vi "Interpret Q Size.vi"(7 "Access":T1, 9 "Waveform Data References":i32[](array[numeric]), 11 "Communication Properties":T2={"WPL"={"Custom Queue Size"=1, "Use Custom Queue Size?"=FALSE}}) -> (1 "Waveform Data References dup":i32[](array[numeric]), 3 "Queue Size":i32=1, 6 "Access dup":T1)   [LabVIEW 2020, in "Internal Comm Classes.lvlib" / "WPL Comm.lvclass"]
uses:
  WPL Comm.lvclass
  Communication Properties.ctl
  Access mode.ctl
  NI_VS Custom Device Waveform API.lvlib
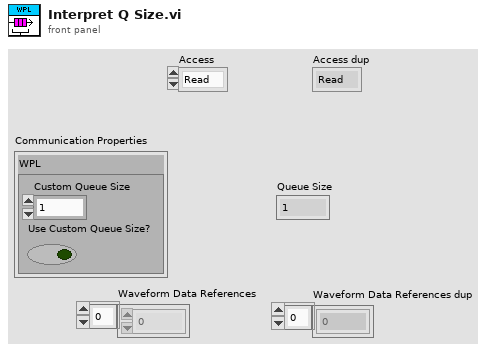
[diagram p1: front panel]
types:
  T1 = typedef "NI_VS Custom Device Waveform API.lvlib/Access mode.ctl" = enum16{"Read", "Write"}
  T2 = typedef "NI_VS Custom Device Waveform API.lvlib/Communication Properties.ctl" = cluster{"WPL":cluster{"Custom Queue Size":i32, "Use Custom Queue Size?":bool}}
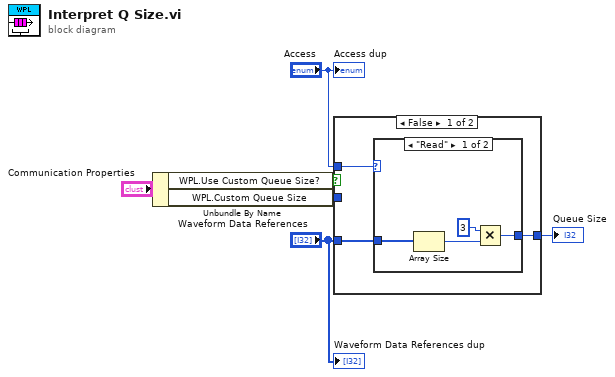
[diagram p0: block diagram]
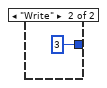
[diagram p2: hidden frame]
diagram:
  n1 = Unbundle By Name("Communication Properties") -> ("WPL.Use Custom Queue Size?"=w5:bool, "WPL.Custom Queue Size"=w3:i32)
  n2 = case shown="False" w5 {
    tunnel: [w7 w15] -> w4
    tunnel: w3 -> [_ w15]
    tunnel: "Access" -> [w9 _]
    tunnel: "Waveform Data References" -> [w8 _]
    frame False {
      n3 = case shown="\"Read\"" w9 {
        tunnel: w8 -> [w13 _]
        tunnel: [w11 3] -> w7
        frame "Read" {
          n4 = Array Size(array=w13) -> (size(s)=w12:i32)
          n5 = Multiply(x=3, y=w12) -> (x*y=w11:i32)
        }
        frame "Write" {
        }
      }
    }
    frame True {
    }
  }
  "Queue Size" <- w4
  "Waveform Data References dup" <- "Waveform Data References"
  "Access dup" <- "Access"
